vi "TimedLoopTest.vi"() -> ()   [LabVIEW 2018]
uses:
  <vilib>/Platform/TimedLoop/XDataNode/timing_clust.ctl
  <vilib>/Platform/TimedLoop/XDataNode/nitl_modes.ctl
  <vilib>/Platform/TimedLoop/XDataNode/wakeup.ctl
  <vilib>/platform/TimedLoop/XDataNode/XDataNode.xnode
  <vilib>/Platform/TimedLoop/XDataNode/XDNodeRunTimeDep.lvlib
panel:
  out "Waveform Graph":u32[](graph)=[100, 300, 500, 700, 900, 200, 400, 600, 800, 1000, 3413202102]
  in  "Array":i32[](array[numeric])=[1, 3, 5, 7, 9, 2, 4, 6, 8, 10]
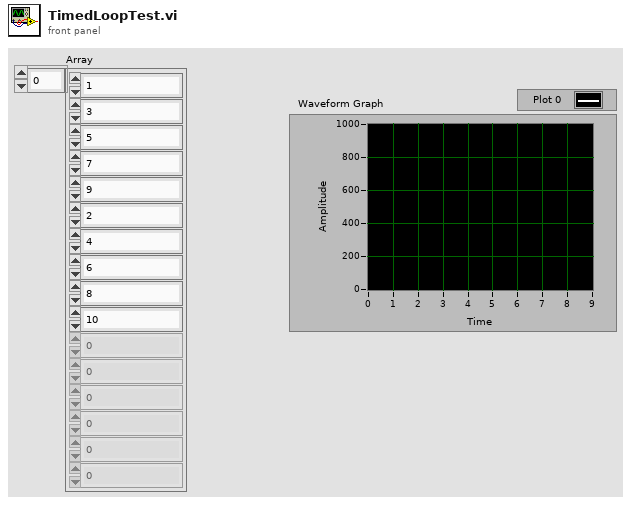
[diagram p1: front panel]
types:
  T1 = typedef "XDNodeRunTimeDep.lvlib/timing_clust.ctl" = cluster{"Expected End [f-1]":u64, "Actual End [f-1]":u64, "Finished Late? [f-1]":bool, "Expected End [i-1]":u64, "Actual End [i-1]":u64, "Finished Late? [i-1]":bool, "Expected Start [i]":u64, "Actual Start [i]":u64, "Expected Start [f]":u64, "Actual Start [f]":u64, "Source Name":string, "Structure Name":string, "Period":i64, "Deadline":i64, "Offset":i64, "Start":i64, "Priority":i32, "Timeout":i32, "Mode":T2, "Wakeup Reason":T3, "Error":errorcluster, "Source Type":string, "Secondary Source Type":string, "Global End Time":u64, "Global Start Time":u64, "Frame Duration":u64, "Iteration Duration":u64, "Assigned CPU":i32, "I/O Scan Engine Mode":u32}
  T2 = typedef "XDNodeRunTimeDep.lvlib/nitl_modes.ctl" = enum32{"No Change", "Process missed periods, maintain original phase", "Discard missed periods, maintain original phase", "Process missed periods, ignore original phase", "Discard missed periods, ignore original phase"}
  T3 = typedef "XDNodeRunTimeDep.lvlib/wakeup.ctl" = enum32{"Normal", "Aborted", "Asynchronous wakeup", "Timing source error", "Timed loop error", "Timeout"}
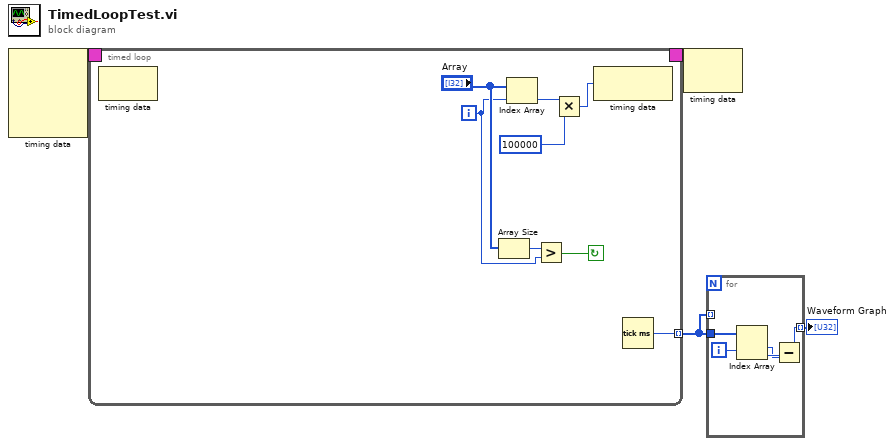
[diagram p0: block diagram]
diagram:
  n1 = node-c288() -> (w4:T1)  [unwired: 4 in]
  n2 = timed-loop {
    timing: w4 -> [_]
    timing-out: [_] -> w3
    tunnel: [w5] -> w1 mode=indexing
    i -> [w7]
    stop <- w6 continue-if-true
    n3 = node-c288() -> ()  [unwired: 1 in, 1 out]
    n4 = Array Size(array="Array") -> (size(s)=w8:i32)
    n5 = Index Array(array="Array", index=w7) -> (element=w12:i32)
    n6 = Greater?(x=w8, y=w7) -> (0:w6:bool)
    n7 = Multiply(x=w12, y=100000) -> (x*y=w11:i32)
    n8 = node-c288(w11) -> ()  [unwired: 1 out]
    n9 = Tick Count (ms)() -> (millisecond timer value=w5:u32)
  }
  n10 = node-c288(w3) -> ()  [unwired: 1 out]
  n11 = for {
    tunnel: w1 -> [w20]
    tunnel: [w17] -> w2 mode=indexing
    tunnel: w1 -> [_] mode=indexing
    i -> [w21]
    n12 = Index Array(array=w20, index #1=w21) -> (element #1=w18:u32, element #2=w19:u32)  [unwired: 1 in]
    n13 = Subtract(x=w19, y=w18) -> (x-y=w17:u32)
  }
  "Waveform Graph" <- w2
